vi "Boiler Controller.vi"(8 "error in":errorcluster, 10 "Notifiers":T1, 11 "Message Queues":T2) -> (0 "error out":errorcluster)   [LabVIEW 2014]
uses:
  support/Message Queue/All Message Queues.ctl
  support/Message Queue/Message Cluster.ctl
  support/Notifiers/Notifiers.ctl
  support/Message Queue/Message Queue.lvlib
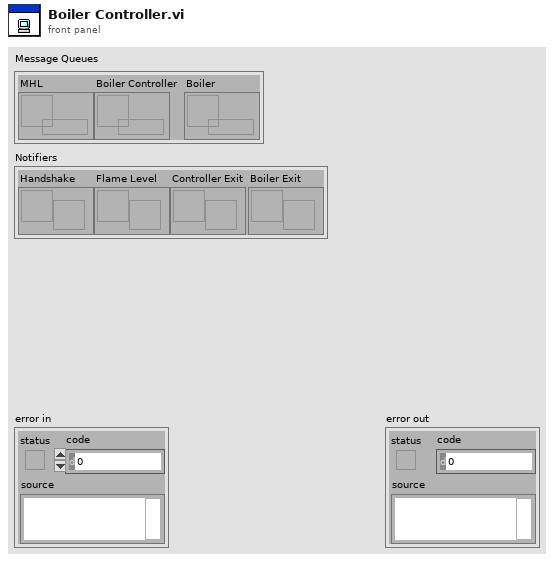
[diagram p1: front panel]
types:
  T1 = typedef "Notifiers.ctl" = cluster{"Handshake":refnum<notifier>, "Flame Level":refnum<notifier>, "Controller Exit":refnum<notifier>, "Boiler Exit":refnum<notifier>}
  T2 = typedef "Message Queue.lvlib/All Message Queues.ctl" = cluster{"MHL":refnum<queue>, "Boiler Controller":refnum<queue>, "Boiler":refnum<queue>}
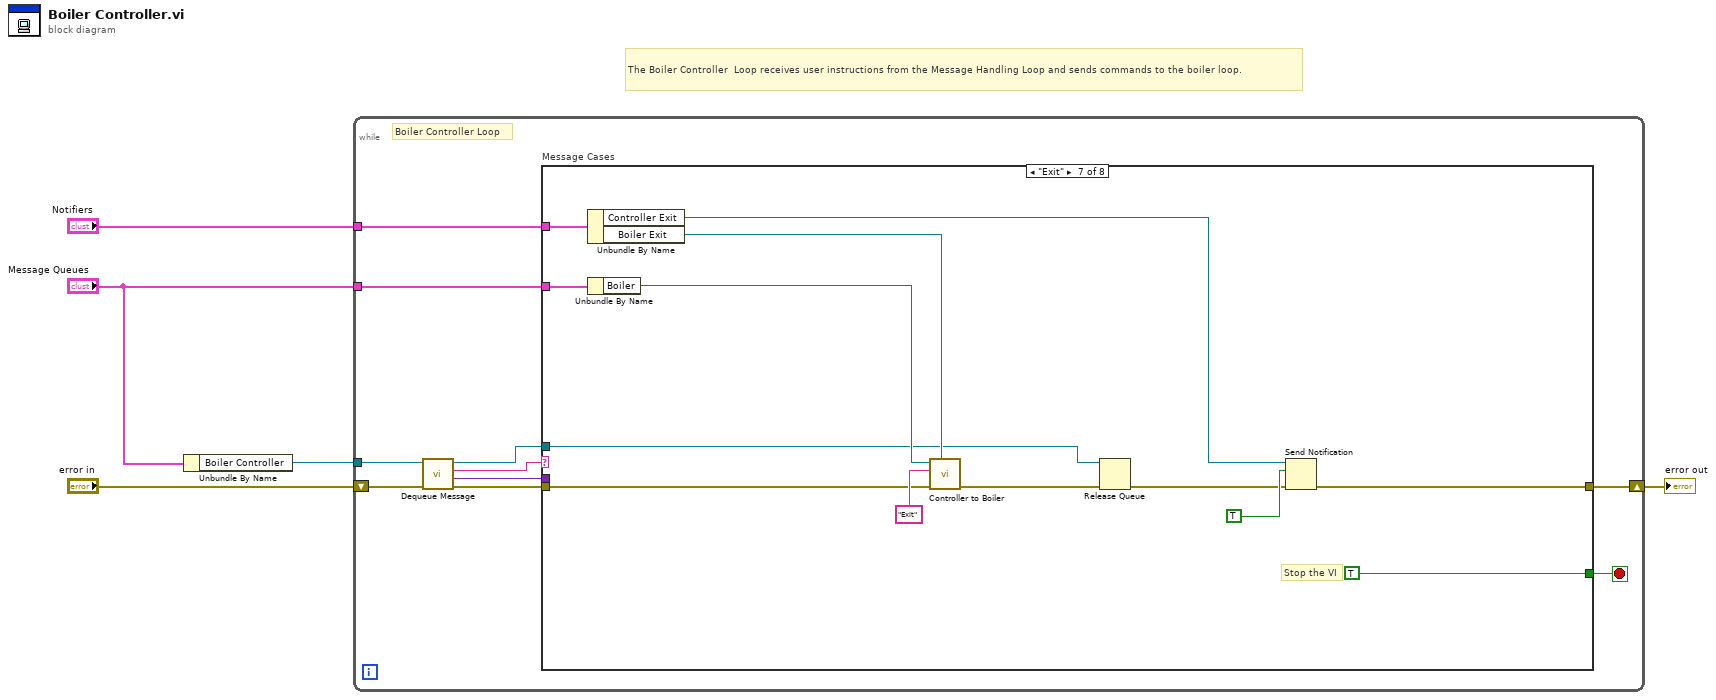
[diagram p0: block diagram]
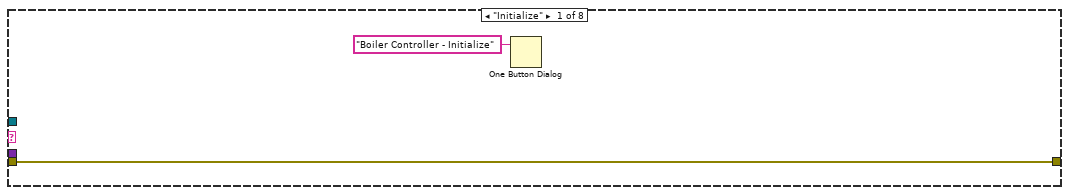
[diagram p2: hidden frame]
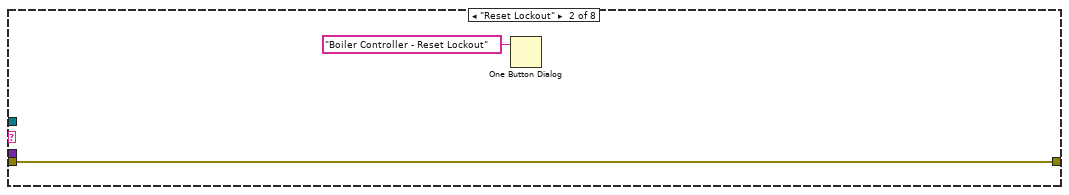
[diagram p3: hidden frame]
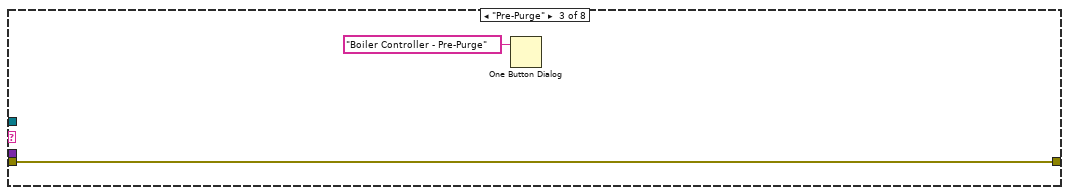
[diagram p4: hidden frame]
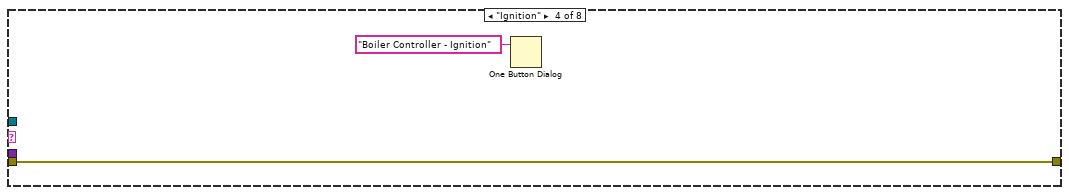
[diagram p5: hidden frame]
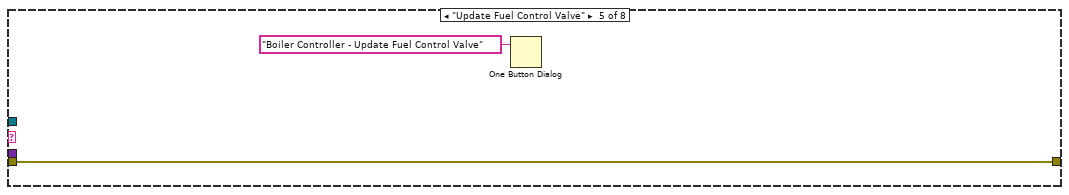
[diagram p6: hidden frame]
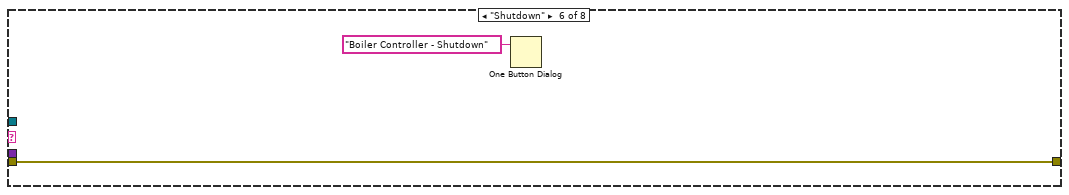
[diagram p7: hidden frame]
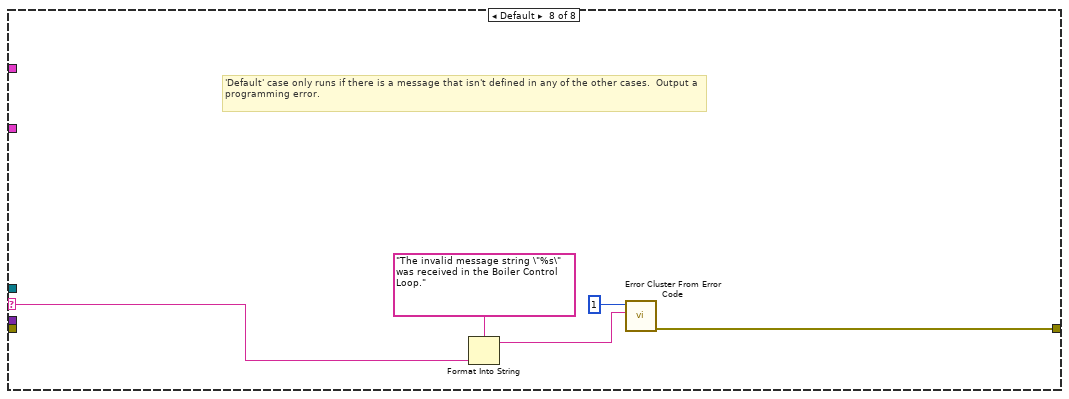
[diagram p8: hidden frame]
diagram:
  # "The Boiler Controller  Loop receives user instructions from the Message Handling Loop and sends commands to the boiler loop."
  n1 = Unbundle By Name("Message Queues") -> ("Boiler Controller"=w3:refnum<queue>)
  n2 = while {
    tunnel: w3 -> [w9]
    shift-right: [w8] -> w5
    shift-left: "error in" -> [w14]
    tunnel: "Message Queues" -> [w7]
    tunnel: "Notifiers" -> [w6]
    stop <- w15 stop-if-true
    # "Boiler Controller Loop"
    n3 = call "Dequeue Message.vi"("error in (no error)"=w14, "Message Queue"=w9) -> ("error out"=w13:errorcluster, "Message Data"=w11:variant, "Message"=w12:string, "dup Message Queue"=w10:refnum<queue>)  [unwired: 6 in]
    n4 = case "Message Cases" shown="\"Exit\"" w12 {
      selector: w12 -> [_ _ _ _ _ _ _ w42]
      tunnel: w10 -> [_ _ _ _ _ _ w33 _]
      tunnel: w13 -> [w17 w19 w21 w23 w25 w27 w32 _]
      tunnel: [w17 w19 w21 w23 w25 w27 w30 w41] -> w8
      tunnel: [_ _ _ _ _ _ TRUE _] -> w15
      tunnel: w11 -> [_ _ _ _ _ _ _ _]
      tunnel: w7 -> [_ _ _ _ _ _ w29 _]
      tunnel: w6 -> [_ _ _ _ _ _ w28 _]
      frame "Initialize" {
        n5 = One Button Dialog(message="Boiler Controller - Initialize") -> ()  [unwired: 1 in, 1 out]
      }
      frame "Reset Lockout" {
        n6 = One Button Dialog(message="Boiler Controller - Reset Lockout") -> ()  [unwired: 1 in, 1 out]
      }
      frame "Pre-Purge" {
        n7 = One Button Dialog(message="Boiler Controller - Pre-Purge") -> ()  [unwired: 1 in, 1 out]
      }
      frame "Ignition" {
        n8 = One Button Dialog(message="Boiler Controller - Ignition") -> ()  [unwired: 1 in, 1 out]
      }
      frame "Update Fuel Control Valve" {
        n9 = One Button Dialog(message="Boiler Controller - Update Fuel Control Valve") -> ()  [unwired: 1 in, 1 out]
      }
      frame "Shutdown" {
        n10 = One Button Dialog(message="Boiler Controller - Shutdown") -> ()  [unwired: 1 in, 1 out]
      }
      frame "Exit" {
        # "Stop the VI"
        n11 = Unbundle By Name(w28) -> ("Controller Exit"=w35:refnum<notifier>, "Boiler Exit"=w37:refnum<notifier>)
        n12 = Unbundle By Name(w29) -> ("Boiler"=w34:refnum<queue>)
        n13 = call "Controller to Boiler.vi"("Notifier"=w37, "error in"=w32, "Message"="Exit", "Boiler Queue in"=w34) -> ("error out"=w40:errorcluster)  [unwired: 5 in, 2 out]
        n14 = Release Queue(queue=w33, error in (no error)=w40) -> (error out=w36:errorcluster)  [unwired: 1 in, 2 out]
        n15 = Send Notification(notification=TRUE, notifier=w35, error in (no error)=w36) -> (error out=w30:errorcluster)  [unwired: 1 out]
      }
      frame Default {
        # "'Default' case only runs if there is a message that isn't defined in any of the other cases.  Output a programming error."
        n16 = Format Into String(format string="The invalid message string \"%s\" was received in the Boiler Control Loop." ("Unknown Message Error Text"), w42) -> (resulting string=w43:string)  [unwired: 2 in, 1 out]
        n17 = call <vilib>:"Error Cluster From Error Code.vi"("error message (\"\")"=w43, "error code (0)"=1) -> ("error out"=w41:errorcluster)  [unwired: 7 in]
      }
    }
  }
  "error out" <- w5
